vi "G_Estados_Rotativa.vi"() -> ()   [LabVIEW 2020]
panel:
  out "Rotativa":T1
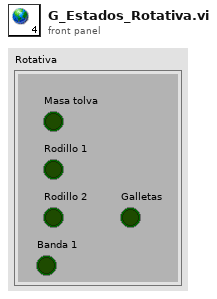
[diagram p1: front panel]
types:
  T1 = cluster{"Masa tolva":bool, "Rodillo 1":bool, "Rodillo 2":bool, "Galletas":bool, "Banda 1":bool}
diagram:
